vi "Signal generation.vi"(7 "system parameters":T2 {"symbol map" format="%.3f"}, 8 "error in (no error)":errorcluster, 9 "filter parameters":T1={"Alpha"=0.5, "Filter Length"=6, "TX Filter"=enum."Root Raised Cos"} {"Alpha" format="%.2f"}, 10 "NumOfSymbols":i32) -> (0 "error out":errorcluster, 1 "pulse shaping filter coefficients":dbl[](array[numeric]) format="%.2f", 2 "input bit stream":i16[](array[numeric]), 3 "output complex waveform":T3 {"Y" format="%.3f"; "dt" format="%^.2e"; "t0" format="%.4f"})   [LabVIEW 2011]
uses:
  <vilib>/addons/Modulation/Analog/controls/Complex Data Waveform.ctl
  FilterCoefficient.ctl
  <vilib>/addons/Modulation/niAMT.lvlib
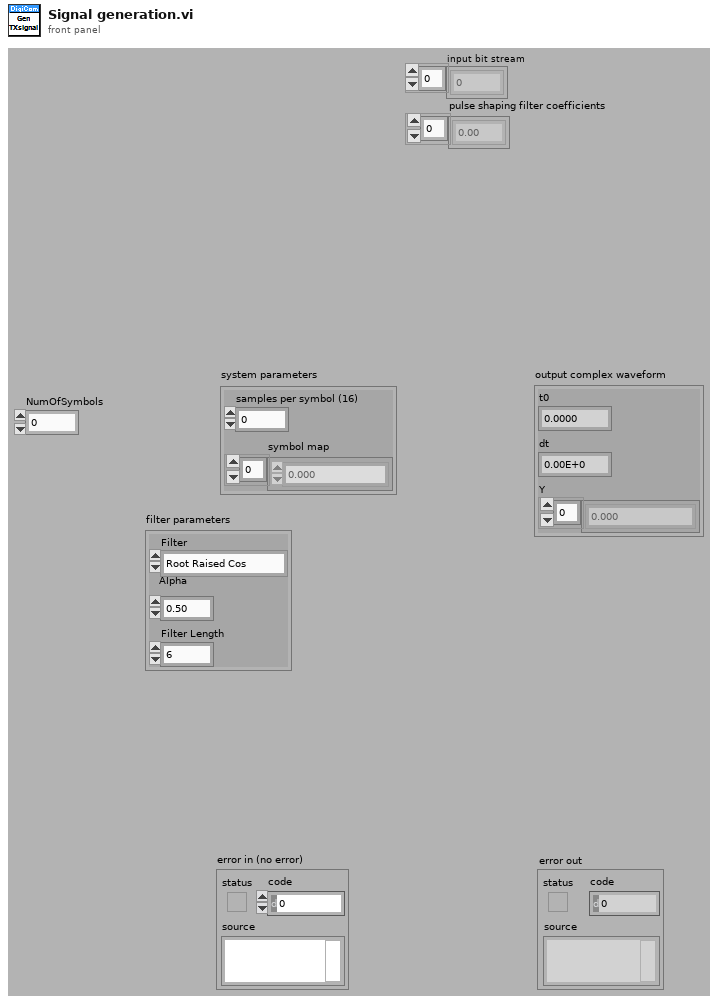
[diagram p1: front panel]
types:
  T1 = typedef "FilterCoefficient.ctl" = cluster{"Alpha":dbl, "Filter Length":i32, "TX Filter":enum16{"Root Raised Cos", "Raised Cos", "Rectangular"}}
  T2 = cluster{"samples per symbol (16)":i32, "symbol map":cdb[]}
  T3 = typedef "niAMT.lvlib/Complex Data Waveform.ctl" = cluster{"t0":dbl, "dt":dbl, "Y":cdb[]}
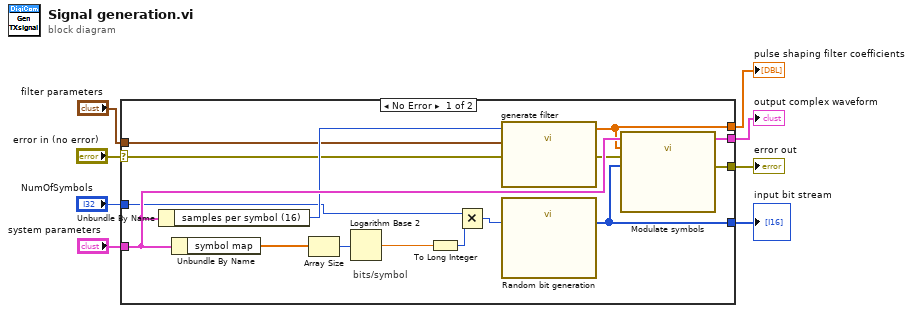
[diagram p0: block diagram]
diagram:
  n1 = case shown="No Error" "error in (no error)" {
    selector: "error in (no error)" -> [w15 w24]
    tunnel: [w12 _] -> w8
    tunnel: [w22 w24] -> w7
    tunnel: "system parameters" -> [w23 _]
    tunnel: "filter parameters" -> [w11 _]
    tunnel: [w13 _] -> w4
    tunnel: "NumOfSymbols" -> [w9 _]
    tunnel: [w10 _] -> w1
    frame No Error {
      # "bits/symbol"
      n2 = Unbundle By Name(w23) -> ("samples per symbol (16)"=w16:i32)
      n3 = Unbundle By Name(w23) -> ("symbol map"=w18:cdb[])
      n4 = Array Size(array=w18) -> (size(s)=w19:i32)
      n5 = Logarithm Base 2(1:w19) -> (0:w20:dbl)
      n6 = To Long Integer(number=w20) -> (32bit integer=w21:i32)
      n7 = Multiply(x=w9, y=w21) -> (x*y=w17:i32)
      n8 = call "generate filter.vi"("error in (no error)"=w15, "filter parameters"=w11, "pulse shaping samples per symbol (16)"=w16) -> ("error out"=w14:errorcluster, "pulse shaping filter coefficients"=w10:dbl[])  [unwired: 6 in, 1 out]
      n9 = call "Random bit generation.vi"("total bits"=w17) -> ("bit stream"=w13:u32[])  [unwired: 10 in]
      n10 = call "Modulate symbols.vi"("input bit stream"=w13, "error in (no error)"=w14, "pulse shaping filter coefficients"=w10, "system parameters"=w23) -> ("error out"=w22:errorcluster, "output complex waveform"=w12:T3)  [unwired: 5 in, 1 out]
    }
    frame Error {
    }
  }
  "error out" <- w7
  "output complex waveform" <- w8
  "input bit stream" <- w4
  "pulse shaping filter coefficients" <- w1
